vi "多参数全局变量.vi"() -> ()   [LabVIEW 2016, in "斯坦道多参数.lvlib"]
uses:
  <vilib>/Plasmionique/MB Master/MB_Master_Serial/MB_Master_Serial.lvclass
panel:
  out "多参数运行状态":u16(ring) items=["空闲", "水样测试", "标样核查"]
  in  "MB_Serial session":refnum<class "MB_Master_Serial.lvclass">
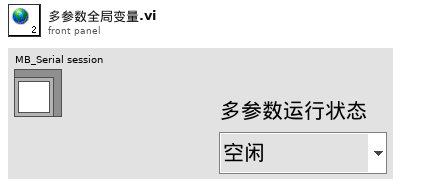
[diagram p1: front panel]
diagram:
